vi "Get VI BD Data.vi"(8 "error in (no error)":errorcluster, 11 "VI ref in":refnum<vi>) -> (0 "error out":errorcluster, 1 "Diagram to Structure":T1, 2 "Structure to Diagram":T5, 3 "VI ref out":refnum<vi>, 5 "BD":T2)   [LabVIEW 2019]
uses:
  <vilib>/Utility/miscctls.llb/LVPositionTypeDef.ctl
  <vilib>/Utility/miscctls.llb/LVBoundsTypeDef.ctl
  Typedefs/BD Data.ctl
  <vilib>/Utility/traverseref.llb/TRef TravTarget.ctl
  <vilib>/Utility/traverseref.llb/VI Scripting - Traverse.lvlib
  <vilib>/Utility/miscctls.llb/LVMapReplaceAction.ctl
  Typedefs/Diagram Group.ctl
  Typedefs/Structure to Diagram.ctl
  Typedefs/Diagram to Structure.ctl
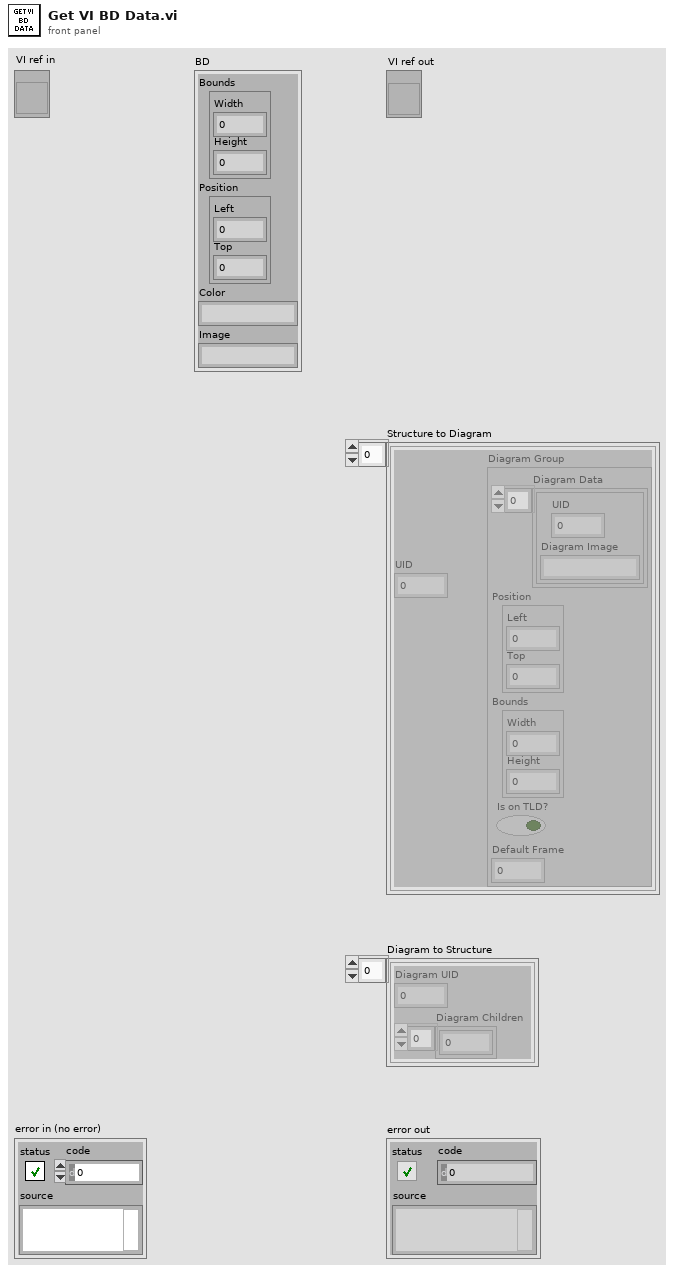
[diagram p1: front panel]
types:
  T1 = typedef "Diagram to Structure.ctl" = cluster{"Diagram UID":i32, "Diagram Children":i32[]}[]
  T2 = typedef "BD Data.ctl" = cluster{"Bounds":T3, "Position":T4, "Color":string, "Image":string}
  T3 = typedef "LVBoundsTypeDef.ctl" = cluster{"Width":u32, "Height":u32}
  T4 = typedef "LVPositionTypeDef.ctl" = cluster{"Left":i32, "Top":i32}
  T5 = typedef "Structure to Diagram.ctl" = cluster{"UID":i32, "Diagram Group":T6}[]
  T6 = typedef "Diagram Group.ctl" = cluster{"Diagram Data":cluster{"UID":i32, "Diagram Image":string}[], "Position":T4, "Bounds":T3, "Is on TLD?":bool, "Default Frame":u32}
  T7 = typedef "TRef TravTarget.ctl" = enum16{"FP", "BD", "Other"}
  T8 = typedef "imagedata.ctl" = cluster{"image type":i32, "image depth":i32, "image":u8[], "mask":u8[], "colors":u32[], "Rectangle":cluster{"left":i16, "top":i16, "right":i16, "bottom":i16}}
  T9 = typedef "LVMapReplaceAction.ctl" = enum32{"Modify Entry only if found", "Add or Modify Entry", "Delete Entry"}
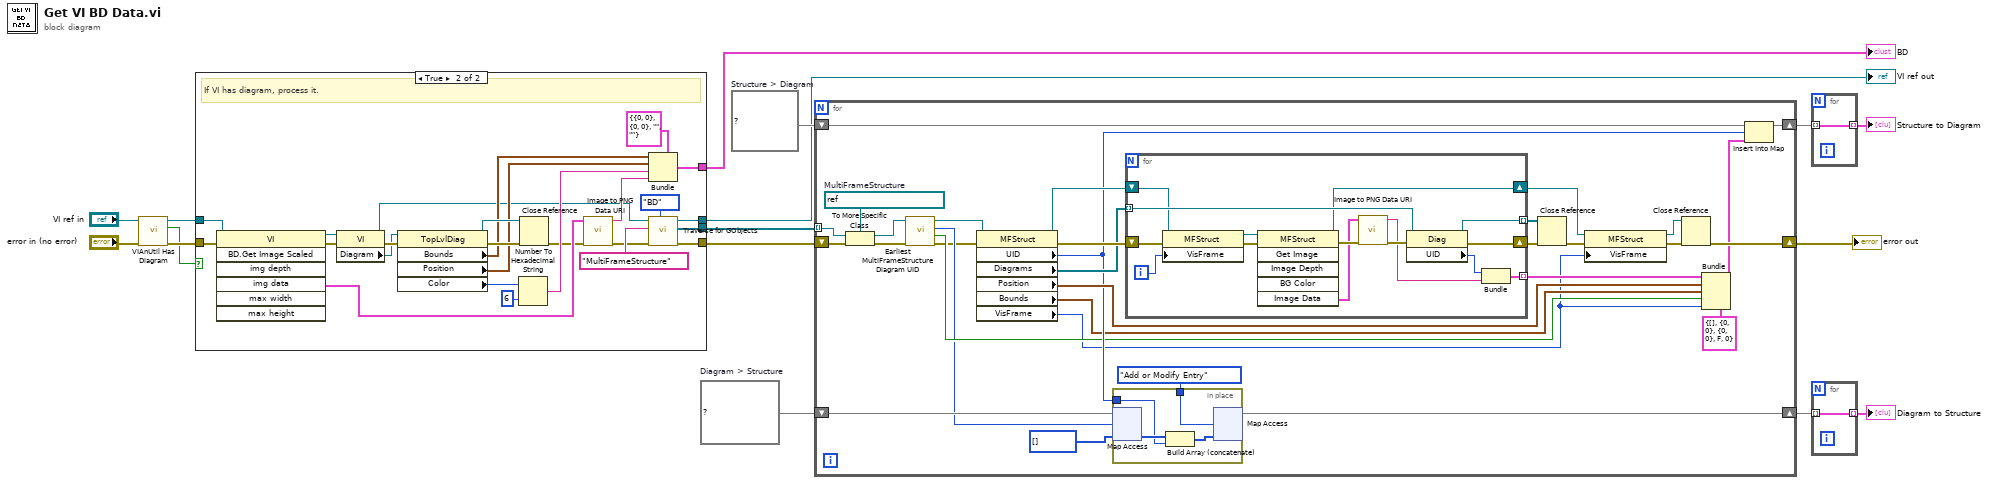
[diagram p0: block diagram]
diagram:
  w12 = map{i32, i32[]} {}  # Diagram > Structure
  w13 = map{i32, T6} {}  # Structure > Diagram
  n1 = call <vilib>:"VIAnUtil Has Diagram.vi"("error in (no error)"="error in (no error)", "VI in"="VI ref in") -> ("error out"=w10:errorcluster, "Has Diag?"=w9:bool, "VI out"=w11:refnum<vi>)  [unwired: 4 in, 3 out]
  n2 = case shown="True" w9 {
    tunnel: [w18 w22] -> w6
    tunnel: [_ w31] -> w3
    tunnel: w11 -> [w17 w28]
    tunnel: w10 -> [w18 w27]
    tunnel: [_ w23] -> w8
    tunnel: [w17 w21] -> w7
    frame False {
      # "If VI does not have diagram (global, control, etc...), skip.\nTool will then show the result as empty block diagram."
    }
    frame True {
      # "If VI has diagram, process it."
      n3 = invoke class="VI" method="BD.Get Image Scaled"(reference=w28, error in=w27) -> (reference out=w42:refnum<vi>, error out=w43:errorcluster, "img data"=w30:T8)  [unwired: 5 in, 4 out]
      n4 = property class="VI"(reference=w42, error in=w43) -> (reference out=w24:refnum<vi>, error out=w41:errorcluster, "Diagram"=w40:refnum<vi>)
      n5 = property class="TopLvlDiag"(reference=w40, error in=w41) -> (reference out=w38:refnum<vi>, error out=w39:errorcluster, "Bounds"=w34:T3, "Position"=w33:T4, "Color"=w36:u32)
      n6 = Number To Hexadecimal String(1:i16 6 ("width (-)"), 2:w36) -> (0:w32:string)
      n7 = Close Reference(reference=w38, error in (no error)=w39) -> (error out=w19:errorcluster)
      n8 = call "Image to PNG Data URI.vi"("error in (no error)"=w19, "Image data"=w30) -> ("error out"=w20:errorcluster, "Base64 encoded"=w29:string)  [unwired: 7 in, 1 out]
      n9 = Bundle(cluster=T2 {"Bounds"={"Width"=0, "Height"=0}, "Position"={"Left"=0, "Top"=0}, "Color"="", "Image"=""} ("BD"), "Bounds"=w34, "Position"=w33, "Color"=w32, "Image"=w29) -> (w31:T2)
      n10 = call <vilib>:"Traverse for GObjects.vi"("Traverse Target"=TRef_TravTarget."BD", "error in (no error)"=w20, "Class Name"="MultiFrameStructure", "VI Refnum"=w24) -> ("error out"=w22:errorcluster, "References"=w23:refnum<vi>[], "dup VI Refnum"=w21:refnum<vi>)  [unwired: 4 in, 1 out]
    }
  }
  "BD" <- w3
  "VI ref out" <- w7
  n11 = for {
    tunnel: w8 -> [w73] mode=indexing
    shift-right: [w68] -> w15
    shift-left: w13 -> [w69]
    shift-right: [w65] -> w16
    shift-left: w6 -> [w74]
    shift-right: [w58] -> w14
    shift-left: w12 -> [w59]
    w72 = refnum<vi> refnum  # MultiFrameStructure
    n12 = To More Specific Class(target class=w72, reference=w73, error in=w74) -> (specific class reference=w49:refnum<vi>, error out=w51:errorcluster)
    n13 = call "Earliest MultiFrameStructure Diagram UID.vi"("error in (no error)"=w51, "MFS ref in"=w49) -> ("error out"=w50:errorcluster, "TLD?"=w53:bool, "UID"=w52:i32, "MFS ref out"=w48:refnum<vi>)  [unwired: 6 in]
    n14 = property class="MFStruct"(reference=w48, error in=w50) -> (reference out=w64:refnum<vi>, error out=w71:errorcluster, "UID"=w56:i32, "Diagrams"=w70:refnum<vi>[], "Position"=w63:T4, "Bounds"=w54:T3, "VisFrame"=w44:u32)
    n15 = in-place {
      in-place-border: LVMapReplaceAction."Add or Modify Entry" ("Replace Action") -> [w76]
      in-place-border: w56 -> [w75]
      n16 = in-place-map #1(w59, w52, i32[] [] ("output cluster")) -> (w78:i32[])  [unwired: 1 out]
      n17 = Build Array (concatenate)(w78, w75) -> (w77:i32[])
      n18 = in-place-map #1(w77, w76) -> (w58:map{i32, i32[]})  [unwired: 2 out]
    }
    n19 = for {
      tunnel: w70 -> [w93] mode=indexing
      tunnel: [w84] -> w62 mode=indexing
      shift-right: [w92] -> w67
      shift-left: w71 -> [w90]
      tunnel: [w91] -> w66 mode=indexing
      shift-right: [w79] -> w46
      shift-left: w64 -> [w89]
      i -> [w88]
      n20 = property class="MFStruct"(reference=w89, error in=w90, "VisFrame"=w88) -> (reference out=w86:refnum<vi>, error out=w87:errorcluster)
      n21 = invoke class="MFStruct" method="Get Image"(reference=w86, error in=w87) -> (reference out=w79:refnum<vi>, error out=w83:errorcluster, "Image Data"=w81:T8)  [unwired: 4 in, 3 out]
      n22 = call "Image to PNG Data URI.vi"("error in (no error)"=w83, "Image data"=w81) -> ("error out"=w82:errorcluster, "Base64 encoded"=w80:string)  [unwired: 7 in, 1 out]
      n23 = property class="Diag"(reference=w93, error in=w82) -> (reference out=w91:refnum<vi>, error out=w92:errorcluster, "UID"=w85:i32)
      n24 = Bundle("UID"=w85, "Base64 encoded"=w80) -> (w84:cluster{"UID":i32, "Base64 encoded":string})  [unwired: 1 in]
    }
    n25 = Close Reference(reference=w66, error in (no error)=w67) -> (error out=w47:errorcluster)
    n26 = property class="MFStruct"(reference=w46, "VisFrame"=w44) -> (reference out=w45:refnum<vi>)  [unwired: 1 in, 1 out]
    n27 = Close Reference(reference=w45, error in (no error)=w47) -> (error out=w65:errorcluster)
    n28 = Bundle(cluster=T6 {"Diagram Data"=[], "Position"={"Left"=0, "Top"=0}, "Bounds"={"Width"=0, "Height"=0}, "Is on TLD?"=FALSE, "Default Frame"=0} ("Diagram Group"), "Diagram Data"=w62, "Position"=w63, "Bounds"=w54, "Is on TLD?"=w53, "Default Frame"=w44) -> (w61:T6)
    n29 = Insert Into Map(map in=w69, key=w56, value=w61) -> (map out=w68:map{i32, T6})  [unwired: 2 out]
  }
  "error out" <- w16
  n30 = for {
    tunnel: w15 -> [w94] mode=indexing
    tunnel: [w94] -> w1 mode=indexing
  }
  "Structure to Diagram" <- w1
  n31 = for {
    tunnel: w14 -> [w95] mode=indexing
    tunnel: [w95] -> w2 mode=indexing
  }
  "Diagram to Structure" <- w2
